vi "App - analyze RUS V6.vi"() -> ()   [LabVIEW 2021] (continued)
"z (pi/2)"=0.0+0.0i, "z center"=0.0+0.0i, "z(0)"=0.0+0.0i, "radius"=0.0}}, "timestamp(min)"=2847.0166666656733, "timestamp"=timestamp(3493898642 s since 1904-01-01), "Magn Field(T)"=0.0}, {"temperature"=14.778, "lorentzian"={"A (VHz)"=0.0, "ω (Hz)"=0.0, "Γ (Hz)"=0.0, "φ (rad)"=0.0, "Q"=0.0, "Norm  Ampl"=0.0, "z∞ (V)"=0.0+0.0i, "4corners"={"z (-pi/2)"=0.0+0.0i, "z(inf)"=0.0+0.0i, "z (pi/2)"=0.0+0.0i, "z center"=0.0+0.0i, "z(0)"=0.0+0.0i, "radius"=0.0}}, "timestamp(min)"=2848.333333335817, "timestamp"=timestamp(3493898721 s since 1904-01-01), "Magn Field(T)"=0.0}, {"temperature"=14.778, "lorentzian"={"A (VHz)"=0.0, "ω (Hz)"=0.0, "Γ (Hz)"=0.0, "φ (rad)"=0.0, "Q"=0.0, "Norm  Ampl"=0.0, "z∞ (V)"=0.0+0.0i, "4corners"={"z (-pi/2)"=0.0+0.0i, "z(inf)"=0.0+0.0i, "z (pi/2)"=0.0+0.0i, "z center"=0.0+0.0i, "z(0)"=0.0+0.0i, "radius"=0.0}}, "timestamp(min)"=2849.666666664183, "timestamp"=timestamp(3493898801 s since 1904-01-01), "Magn Field(T)"=0.0}, {"temperature"=14.784, "lorentzian"={"A (VHz)"=0.0, "ω (Hz)"=0.0, "Γ (Hz)"=0.0, "φ (rad)"=0.0, "Q"=0.0, "Norm  Ampl"=0.0, "z∞ (V)"=0.0+0.0i, "4corners"={"z (-pi/2)"=0.0+0.0i, "z(inf)"=0.0+0.0i, "z (pi/2)"=0.0+0.0i, "z center"=0.0+0.0i, "z(0)"=0.0+0.0i, "radius"=0.0}}, "timestamp(min)"=2850.9833333343267, "timestamp"=timestamp(3493898880 s since 1904-01-01), "Magn Field(T)"=0.0}, {"temperature"=14.784, "lorentzian"={"A (VHz)"=0.0, "ω (Hz)"=0.0, "Γ (Hz)"=0.0, "φ (rad)"=0.0, "Q"=0.0, "Norm  Ampl"=0.0, "z∞ (V)"=0.0+0.0i, "4corners"={"z (-pi/2)"=0.0+0.0i, "z(inf)"=0.0+0.0i, "z (pi/2)"=0.0+0.0i, "z center"=0.0+0.0i, "z(0)"=0.0+0.0i, "radius"=0.0}}, "timestamp(min)"=2852.3000000044703, "timestamp"=timestamp(3493898959 s since 1904-01-01), "Magn Field(T)"=0.0}, {"temperature"=14.784, "lorentzian"={"A (VHz)"=0.0, "ω (Hz)"=0.0, "Γ (Hz)"=0.0, "φ (rad)"=0.0, "Q"=0.0, "Norm  Ampl"=0.0, "z∞ (V)"=0.0+0.0i, "4corners"={"z (-pi/2)"=0.0+0.0i, "z(inf)"=0.0+0.0i, "z (pi/2)"=0.0+0.0i, "z center"=0.0+0.0i, "z(0)"=0.0+0.0i, "radius"=0.0}}, "timestamp(min)"=2853.6333333328366, "timestamp"=timestamp(3493899039 s since 1904-01-01), "Magn Field(T)"=0.0}, {"temperature"=14.789, "lorentzian"={"A (VHz)"=0.0, "ω (Hz)"=0.0, "Γ (Hz)"=0.0, "φ (rad)"=0.0, "Q"=0.0, "Norm  Ampl"=0.0, "z∞ (V)"=0.0+0.0i, "4corners"={"z (-pi/2)"=0.0+0.0i, "z(inf)"=0.0+0.0i, "z (pi/2)"=0.0+0.0i, "z center"=0.0+0.0i, "z(0)"=0.0+0.0i, "radius"=0.0}}, "timestamp(min)"=2854.9500000029802, "timestamp"=timestamp(3493899118 s since 1904-01-01), "Magn Field(T)"=0.0}, {"temperature"=14.788, "lorentzian"={"A (VHz)"=0.0, "ω (Hz)"=0.0, "Γ (Hz)"=0.0, "φ (rad)"=0.0, "Q"=0.0, "Norm  Ampl"=0.0, "z∞ (V)"=0.0+0.0i, "4corners"={"z (-pi/2)"=0.0+0.0i, "z(inf)"=0.0+0.0i, "z (pi/2)"=0.0+0.0i, "z center"=0.0+0.0i, "z(0)"=0.0+0.0i, "radius"=0.0}}, "timestamp(min)"=2856.2833333313465, "timestamp"=timestamp(3493899198 s since 1904-01-01), "Magn Field(T)"=0.0}, {"temperature"=14.791, "lorentzian"={"A (VHz)"=0.0, "ω (Hz)"=0.0, "Γ (Hz)"=0.0, "φ (rad)"=0.0, "Q"=0.0, "Norm  Ampl"=0.0, "z∞ (V)"=0.0+0.0i, "4corners"={"z (-pi/2)"=0.0+0.0i, "z(inf)"=0.0+0.0i, "z (pi/2)"=0.0+0.0i, "z center"=0.0+0.0i, "z(0)"=0.0+0.0i, "radius"=0.0}}, "timestamp(min)"=2857.60000000149, "timestamp"=timestamp(3493899277 s since 1904-01-01), "Magn Field(T)"=0.0}, {"temperature"=14.793, "lorentzian"={"A (VHz)"=0.0, "ω (Hz)"=0.0, "Γ (Hz)"=0.0, "φ (rad)"=0.0, "Q"=0.0, "Norm  Ampl"=0.0, "z∞ (V)"=0.0+0.0i, "4corners"={"z (-pi/2)"=0.0+0.0i, "z(inf)"=0.0+0.0i, "z (pi/2)"=0.0+0.0i, "z center"=0.0+0.0i, "z(0)"=0.0+0.0i, "radius"=0.0}}, "timestamp(min)"=2858.916666664183, "timestamp"=timestamp(3493899356 s since 1904-01-01), "Magn Field(T)"=0.0}, {"temperature"=14.796, "lorentzian"={"A (VHz)"=0.0, "ω (Hz)"=0.0, "Γ (Hz)"=0.0, "φ (rad)"=0.0, "Q"=0.0, "Norm  Ampl"=0.0, "z∞ (V)"=0.0+0.0i, "4corners"={"z (-pi/2)"=0.0+0.0i, "z(inf)"=0.0+0.0i, "z (pi/2)"=0.0+0.0i, "z center"=0.0+0.0i, "z(0)"=0.0+0.0i, "radius"=0.0}}, "timestamp(min)"=2860.25, "timestamp"=timestamp(3493899436 s since 1904-01-01), "Magn Field(T)"=0.0}, {"temperature"=14.797, "lorentzian"={"A (VHz)"=0.0, "ω (Hz)"=0.0, "Γ (Hz)"=0.0, "φ (rad)"=0.0, "Q"=0.0, "Norm  Ampl"=0.0, "z∞ (V)"=0.0+0.0i, "4corners"={"z (-pi/2)"=0.0+0.0i, "z(inf)"=0.0+0.0i, "z (pi/2)"=0.0+0.0i, "z center"=0.0+0.0i, "z(0)"=0.0+0.0i, "radius"=0.0}}, "timestamp(min)"=2861.5666666701436, "timestamp"=timestamp(3493899515 s since 1904-01-01), "Magn Field(T)"=0.0}, {"temperature"=14.8, "lorentzian"={"A (VHz)"=0.0, "ω (Hz)"=0.0, "Γ (Hz)"=0.0, "φ (rad)"=0.0, "Q"=0.0, "Norm  Ampl"=0.0, "z∞ (V)"=0.0+0.0i, "4corners"={"z (-pi/2)"=0.0+0.0i, "z(inf)"=0.0+0.0i, "z (pi/2)"=0.0+0.0i, "z center"=0.0+0.0i, "z(0)"=0.0+0.0i, "radius"=0.0}}, "timestamp(min)"=2862.8833333328366, "timestamp"=timestamp(3493899594 s since 1904-01-01), "Magn Field(T)"=0.0}, {"temperature"=14.807, "lorentzian"={"A (VHz)"=0.0, "ω (Hz)"=0.0, "Γ (Hz)"=0.0, "φ (rad)"=0.0, "Q"=0.0, "Norm  Ampl"=0.0, "z∞ (V)"=0.0+0.0i, "4corners"={"z (-pi/2)"=0.0+0.0i, "z(inf)"=0.0+0.0i, "z (pi/2)"=0.0+0.0i, "z center"=0.0+0.0i, "z(0)"=0.0+0.0i, "radius"=0.0}}, "timestamp(min)"=2864.2166666686535, "timestamp"=timestamp(3493899674 s since 1904-01-01), "Magn Field(T)"=0.0}, {"temperature"=14.806, "lorentzian"={"A (VHz)"=0.0, "ω (Hz)"=0.0, "Γ (Hz)"=0.0, "φ (rad)"=0.0, "Q"=0.0, "Norm  Ampl"=0.0, "z∞ (V)"=0.0+0.0i, "4corners"={"z (-pi/2)"=0.0+0.0i, "z(inf)"=0.0+0.0i, "z (pi/2)"=0.0+0.0i, "z center"=0.0+0.0i, "z(0)"=0.0+0.0i, "radius"=0.0}}, "timestamp(min)"=2865.5333333313465, "timestamp"=timestamp(3493899753 s since 1904-01-01), "Magn Field(T)"=0.0}, {"temperature"=14.808, "lorentzian"={"A (VHz)"=0.0, "ω (Hz)"=0.0, "Γ (Hz)"=0.0, "φ (rad)"=0.0, "Q"=0.0, "Norm  Ampl"=0.0, "z∞ (V)"=0.0+0.0i, "4corners"={"z (-pi/2)"=0.0+0.0i, "z(inf)"=0.0+0.0i, "z (pi/2)"=0.0+0.0i, "z center"=0.0+0.0i, "z(0)"=0.0+0.0i, "radius"=0.0}}, "timestamp(min)"=2866.8666666671634, "timestamp"=timestamp(3493899833 s since 1904-01-01), "Magn Field(T)"=0.0}, {"temperature"=14.812, "lorentzian"={"A (VHz)"=0.0, "ω (Hz)"=0.0, "Γ (Hz)"=0.0, "φ (rad)"=0.0, "Q"=0.0, "Norm  Ampl"=0.0, "z∞ (V)"=0.0+0.0i, "4corners"={"z (-pi/2)"=0.0+0.0i, "z(inf)"=0.0+0.0i, "z (pi/2)"=0.0+0.0i, "z center"=0.0+0.0i, "z(0)"=0.0+0.0i, "radius"=0.0}}, "timestamp(min)"=2868.183333337307, "timestamp"=timestamp(3493899912 s since 1904-01-01), "Magn Field(T)"=0.0}, {"temperature"=14.814, "lorentzian"={"A (VHz)"=0.0, "ω (Hz)"=0.0, "Γ (Hz)"=0.0, "φ (rad)"=0.0, "Q"=0.0, "Norm  Ampl"=0.0, "z∞ (V)"=0.0+0.0i, "4corners"={"z (-pi/2)"=0.0+0.0i, "z(inf)"=0.0+0.0i, "z (pi/2)"=0.0+0.0i, "z center"=0.0+0.0i, "z(0)"=0.0+0.0i, "radius"=0.0}}, "timestamp(min)"=2869.5, "timestamp"=timestamp(3493899991 s since 1904-01-01), "Magn Field(T)"=0.0}, {"temperature"=14.82, "lorentzian"={"A (VHz)"=0.0, "ω (Hz)"=0.0, "Γ (Hz)"=0.0, "φ (rad)"=0.0, "Q"=0.0, "Norm  Ampl"=0.0, "z∞ (V)"=0.0+0.0i, "4corners"={"z (-pi/2)"=0.0+0.0i, "z(inf)"=0.0+0.0i, "z (pi/2)"=0.0+0.0i, "z center"=0.0+0.0i, "z(0)"=0.0+0.0i, "radius"=0.0}}, "timestamp(min)"=2870.833333335817, "timestamp"=timestamp(3493900071 s since 1904-01-01), "Magn Field(T)"=0.0}, {"temperature"=14.816, "lorentzian"={"A (VHz)"=0.0, "ω (Hz)"=0.0, "Γ (Hz)"=0.0, "φ (rad)"=0.0, "Q"=0.0, "Norm  Ampl"=0.0, "z∞ (V)"=0.0+0.0i, "4corners"={"z (-pi/2)"=0.0+0.0i, "z(inf)"=0.0+0.0i, "z (pi/2)"=0.0+0.0i, "z center"=0.0+0.0i, "z(0)"=0.0+0.0i, "radius"=0.0}}, "timestamp(min)"=2872.14999999851, "timestamp"=timestamp(3493900150 s since 1904-01-01), "Magn Field(T)"=0.0}] {"lorentzian"."z∞ (V)" format="%#_4p"; "lorentzian"."Q" format="%#_4p"; "lorentzian"."φ (rad)" format="%#_3p"; "lorentzian"."Γ (Hz)" format="%#_5p"; "lorentzian"."ω (Hz)" format="%#_9p"; "lorentzian"."A (VHz)" format="%#_3p"}
  in  "cursor bracket: fragment":T24={"left"=663.5468604577721, "right "=663.8468604577721, "center"=663.6968604577721, "window"=0.30000000000000004, "cursors"=[0, 1, 2], "relative"=0, "absolute"=0, "fixed vertical offset"=0.0, "vertical offset"=0.0, "skew"=0.0, "default window frac"=0.1, "kind"=enum."symmetric", "skew.left"=0.5, "skew.right"=0.5, "Plot ref"=refnum, "wing order"=enum."back"}
  in  "cursor bracket: All, data window":T24={"left"=655.6615812868605, "right "=667.1582032202367, "center"=663.6968604577721, "window"=11.496621933376199, "cursors"=[0, 1, 2], "relative"=0, "absolute"=0, "fixed vertical offset"=0.0, "vertical offset"=0.0, "skew"=-0.3978504672897196, "default window frac"=0.1, "kind"=enum."skewed", "skew.left"=0.6989252336448598, "skew.right"=0.3010747663551402, "Plot ref"=refnum, "wing order"=enum."back"}
  in  "cursor bracket: All,  zoom":T24={"left"=842.6955942299186, "right "=2207.477971149593, "center"=1525.0867826897559, "window"=1364.7823769196746, "cursors"=[3, 4, 5], "relative"=0, "absolute"=0, "fixed vertical offset"=0.0, "vertical offset"=0.0, "skew"=0.0, "default window frac"=0.1, "kind"=enum."symmetric", "skew.left"=0.5, "skew.right"=0.5, "Plot ref"=refnum, "wing order"=enum."back"}
  in  "plot scale: Geometry":T28={"Plot Ref"=refnum, "center"=0.0, "delta"=100.0, "mode"=enum."no filter", "scale cursor index"=10, "history"=100.0, "history array"=[0.5, 0.5, 0.5, 0.5, 0.5, 0.5, 0.5, 0.5, 0.5, 0.5, 0.5, 0.5, 0.5, 0.5, 0.5, 0.5, 0.5, 0.5, 0.5, 0.5, 0.5, 0.5, 0.5, 0.5, 0.5, 0.5, 0.5, 0.5, 0.5, 0.5, 0.5, 0.5, 0.5, 0.5, 0.5, 0.5, 0.5, 0.5, 0.5, 0.5, 0.5, 0.5, 0.5, 0.5, 0.5, 0.5, 0.5, 0.5, 0.5, 0.5, 0.5, 0.5, 0.5, 0.5, 0.5, 0.5, 0.5, 0.5, 0.5, 0.5, 0.5, 0.5, 0.5, 0.5, 0.5, 0.5, 0.5, 0.5, 0.5, 0.5, 0.5, 0.5, 0.5, 0.5, 0.5, 0.5, 0.5, 0.5, 0.5, 0.5, 0.5, 0.5, 0.5, 0.5, 0.5, 0.5, 0.5, 0.5, 0.5, 0.5, 0.5, 0.5, 0.5, 0.5, 0.5, 0.5, 0.5, 0.5, 0.5, 0.5]}
  in  "plot scale: delta f":T28={"Plot Ref"=refnum, "center"=0.0, "delta"=60.0, "mode"=enum."no filter", "scale cursor index"=10, "history"=100.0, "history array"=[0.5, 0.5, 0.5, 0.5, 0.5, 0.5, 0.5, 0.5, 0.5, 0.5, 0.5, 0.5, 0.5, 0.5, 0.5, 0.5, 0.5, 0.5, 0.5, 0.5, 0.5, 0.5, 0.5, 0.5, 0.5, 0.5, 0.5, 0.5, 0.5, 0.5, 0.5, 0.5, 0.5, 0.5, 0.5, 0.5, 0.5, 0.5, 0.5, 0.5, 0.5, 0.5, 0.5, 0.5, 0.5, 0.5, 0.5, 0.5, 0.5, 0.5, 0.5, 0.5, 0.5, 0.5, 0.5, 0.5, 0.5, 0.5, 0.5, 0.5, 0.5, 0.5, 0.5, 0.5, 0.5, 0.5, 0.5, 0.5, 0.5, 0.5, 0.5, 0.5, 0.5, 0.5, 0.5, 0.5, 0.5, 0.5, 0.5, 0.5, 0.5, 0.5, 0.5, 0.5, 0.5, 0.5, 0.5, 0.5, 0.5, 0.5, 0.5, 0.5, 0.5, 0.5, 0.5, 0.5, 0.5, 0.5, 0.5, 0.5]}
  in  "plot scale: frequency vs T":T28={"Plot Ref"=refnum, "center"=0.0, "delta"=100.0, "mode"=enum."no filter", "scale cursor index"=10, "history"=100.0, "history array"=[0.5, 0.5, 0.5, 0.5, 0.5, 0.5, 0.5, 0.5, 0.5, 0.5, 0.5, 0.5, 0.5, 0.5, 0.5, 0.5, 0.5, 0.5, 0.5, 0.5, 0.5, 0.5, 0.5, 0.5, 0.5, 0.5, 0.5, 0.5, 0.5, 0.5, 0.5, 0.5, 0.5, 0.5, 0.5, 0.5, 0.5, 0.5, 0.5, 0.5, 0.5, 0.5, 0.5, 0.5, 0.5, 0.5, 0.5, 0.5, 0.5, 0.5, 0.5, 0.5, 0.5, 0.5, 0.5, 0.5, 0.5, 0.5, 0.5, 0.5, 0.5, 0.5, 0.5, 0.5, 0.5, 0.5, 0.5, 0.5, 0.5, 0.5, 0.5, 0.5, 0.5, 0.5, 0.5, 0.5, 0.5, 0.5, 0.5, 0.5, 0.5, 0.5, 0.5, 0.5, 0.5, 0.5, 0.5, 0.5, 0.5, 0.5, 0.5, 0.5, 0.5, 0.5, 0.5, 0.5, 0.5, 0.5, 0.5, 0.5]}
  in  "plot scale: All":T28={"Plot Ref"=refnum, "center"=0.0, "delta"=0.1, "mode"=enum."no filter", "scale cursor index"=10, "history"=100.0, "history array"=[0.5, 0.5, 0.5, 0.5, 0.5, 0.5, 0.5, 0.5, 0.5, 0.5, 0.5, 0.5, 0.5, 0.5, 0.5, 0.5, 0.5, 0.5, 0.5, 0.5, 0.5, 0.5, 0.5, 0.5, 0.5, 0.5, 0.5, 0.5, 0.5, 0.5, 0.5, 0.5, 0.5, 0.5, 0.5, 0.5, 0.5, 0.5, 0.5, 0.5, 0.5, 0.5, 0.5, 0.5, 0.5, 0.5, 0.5, 0.5, 0.5, 0.5, 0.5, 0.5, 0.5, 0.5, 0.5, 0.5, 0.5, 0.5, 0.5, 0.5, 0.5, 0.5, 0.5, 0.5, 0.5, 0.5, 0.5, 0.5, 0.5, 0.5, 0.5, 0.5, 0.5, 0.5, 0.5, 0.5, 0.5, 0.5, 0.5, 0.5, 0.5, 0.5, 0.5, 0.5, 0.5, 0.5, 0.5, 0.5, 0.5, 0.5, 0.5, 0.5, 0.5, 0.5, 0.5, 0.5, 0.5, 0.5, 0.5, 0.5]}
  in  "plot scale: Attenuation vs T":T28={"Plot Ref"=refnum, "center"=0.0, "delta"=50.0, "mode"=enum."no filter", "scale cursor index"=10, "history"=100.0, "history array"=[0.5, 0.5, 0.5, 0.5, 0.5, 0.5, 0.5, 0.5, 0.5, 0.5, 0.5, 0.5, 0.5, 0.5, 0.5, 0.5, 0.5, 0.5, 0.5, 0.5, 0.5, 0.5, 0.5, 0.5, 0.5, 0.5, 0.5, 0.5, 0.5, 0.5, 0.5, 0.5, 0.5, 0.5, 0.5, 0.5, 0.5, 0.5, 0.5, 0.5, 0.5, 0.5, 0.5, 0.5, 0.5, 0.5, 0.5, 0.5, 0.5, 0.5, 0.5, 0.5, 0.5, 0.5, 0.5, 0.5, 0.5, 0.5, 0.5, 0.5, 0.5, 0.5, 0.5, 0.5, 0.5, 0.5, 0.5, 0.5, 0.5, 0.5, 0.5, 0.5, 0.5, 0.5, 0.5, 0.5, 0.5, 0.5, 0.5, 0.5, 0.5, 0.5, 0.5, 0.5, 0.5, 0.5, 0.5, 0.5, 0.5, 0.5, 0.5, 0.5, 0.5, 0.5, 0.5, 0.5, 0.5, 0.5, 0.5, 0.5]}
  in  "9w folder path":path=path "D:/Data/Ultrasound/LSCO/LSCO22__130814c/5_Cooling_2nd_try/9w"
  in  "help toggle":bool=TRUE
  in  "cursor bracket: All,  show":T24={"left"=1443.1667294308304, "right "=1448.993434554408, "center"=1446.0800819926192, "window"=5.826705123577359, "cursors"=[6, 7, 8], "relative"=0, "absolute"=0, "fixed vertical offset"=0.0, "vertical offset"=0.0, "skew"=0.0, "default window frac"=0.1, "kind"=enum."symmetric", "skew.left"=0.5, "skew.right"=0.5, "Plot ref"=refnum, "wing order"=enum."back"}
  in  "plot scale: df/dT":T28={"Plot Ref"=refnum, "center"=0.0, "delta"=60.0, "mode"=enum."no filter", "scale cursor index"=10, "history"=100.0, "history array"=[0.5, 0.5, 0.5, 0.5, 0.5, 0.5, 0.5, 0.5, 0.5, 0.5, 0.5, 0.5, 0.5, 0.5, 0.5, 0.5, 0.5, 0.5, 0.5, 0.5, 0.5, 0.5, 0.5, 0.5, 0.5, 0.5, 0.5, 0.5, 0.5, 0.5, 0.5, 0.5, 0.5, 0.5, 0.5, 0.5, 0.5, 0.5, 0.5, 0.5, 0.5, 0.5, 0.5, 0.5, 0.5, 0.5, 0.5, 0.5, 0.5, 0.5, 0.5, 0.5, 0.5, 0.5, 0.5, 0.5, 0.5, 0.5, 0.5, 0.5, 0.5, 0.5, 0.5, 0.5, 0.5, 0.5, 0.5, 0.5, 0.5, 0.5, 0.5, 0.5, 0.5, 0.5, 0.5, 0.5, 0.5, 0.5, 0.5, 0.5, 0.5, 0.5, 0.5, 0.5, 0.5, 0.5, 0.5, 0.5, 0.5, 0.5, 0.5, 0.5, 0.5, 0.5, 0.5, 0.5, 0.5, 0.5, 0.5, 0.5]}
  in  "plots: filter related":T29
  in  "plot scale: Attenuation vs H":T28={"Plot Ref"=refnum, "center"=0.0, "delta"=50.0, "mode"=enum."no filter", "scale cursor index"=10, "history"=100.0, "history array"=[0.5, 0.5, 0.5, 0.5, 0.5, 0.5, 0.5, 0.5, 0.5, 0.5, 0.5, 0.5, 0.5, 0.5, 0.5, 0.5, 0.5, 0.5, 0.5, 0.5, 0.5, 0.5, 0.5, 0.5, 0.5, 0.5, 0.5, 0.5, 0.5, 0.5, 0.5, 0.5, 0.5, 0.5, 0.5, 0.5, 0.5, 0.5, 0.5, 0.5, 0.5, 0.5, 0.5, 0.5, 0.5, 0.5, 0.5, 0.5, 0.5, 0.5, 0.5, 0.5, 0.5, 0.5, 0.5, 0.5, 0.5, 0.5, 0.5, 0.5, 0.5, 0.5, 0.5, 0.5, 0.5, 0.5, 0.5, 0.5, 0.5, 0.5, 0.5, 0.5, 0.5, 0.5, 0.5, 0.5, 0.5, 0.5, 0.5, 0.5, 0.5, 0.5, 0.5, 0.5, 0.5, 0.5, 0.5, 0.5, 0.5, 0.5, 0.5, 0.5, 0.5, 0.5, 0.5, 0.5, 0.5, 0.5, 0.5, 0.5]}
  in  "plot scale: frequency vs H":T28={"Plot Ref"=refnum, "center"=0.0, "delta"=50.0, "mode"=enum."no filter", "scale cursor index"=10, "history"=100.0, "history array"=[0.5, 0.5, 0.5, 0.5, 0.5, 0.5, 0.5, 0.5, 0.5, 0.5, 0.5, 0.5, 0.5, 0.5, 0.5, 0.5, 0.5, 0.5, 0.5, 0.5, 0.5, 0.5, 0.5, 0.5, 0.5, 0.5, 0.5, 0.5, 0.5, 0.5, 0.5, 0.5, 0.5, 0.5, 0.5, 0.5, 0.5, 0.5, 0.5, 0.5, 0.5, 0.5, 0.5, 0.5, 0.5, 0.5, 0.5, 0.5, 0.5, 0.5, 0.5, 0.5, 0.5, 0.5, 0.5, 0.5, 0.5, 0.5, 0.5, 0.5, 0.5, 0.5, 0.5, 0.5, 0.5, 0.5, 0.5, 0.5, 0.5, 0.5, 0.5, 0.5, 0.5, 0.5, 0.5, 0.5, 0.5, 0.5, 0.5, 0.5, 0.5, 0.5, 0.5, 0.5, 0.5, 0.5, 0.5, 0.5, 0.5, 0.5, 0.5, 0.5, 0.5, 0.5, 0.5, 0.5, 0.5, 0.5, 0.5, 0.5]}
  out "script event":string
  in  "tfolder":T30={"tfolder path"=path "D:/Data/Ultrasound/LSCO/LSCO22__130814c/5_Cooling_2nd_try", "9folder path"=path "D:/Data/Ultrasound/LSCO/LSCO22__130814c/5_Cooling_2nd_try/9w", "tfolder  -  file array"=[{"timestamp from"=43.433333337306976, "timestamp to"=2233.166666664183, " index  from"=17, "index to"=1672, "active"=TRUE}, {"timestamp from"=2241.10000000149, "timestamp to"=2399.8666666671634, " index  from"=1678, "index to"=1798, "active"=TRUE}, {"timestamp from"=2423.683333337307, "timestamp to"=2870.833333335817, " index  from"=1816, "index to"=2154, "active"=TRUE}], "from index array"=[17, 1678, 1816], "timestamp array"=[43.433333337306976, 2241.10000000149, 2423.683333337307]}
  in  "Tab : dummy":enum32{"Page 1", "Page 2"}(tab)
  out "Plot: dTemp/dTime":cluster{dbl[], dbl[]}[](graph)
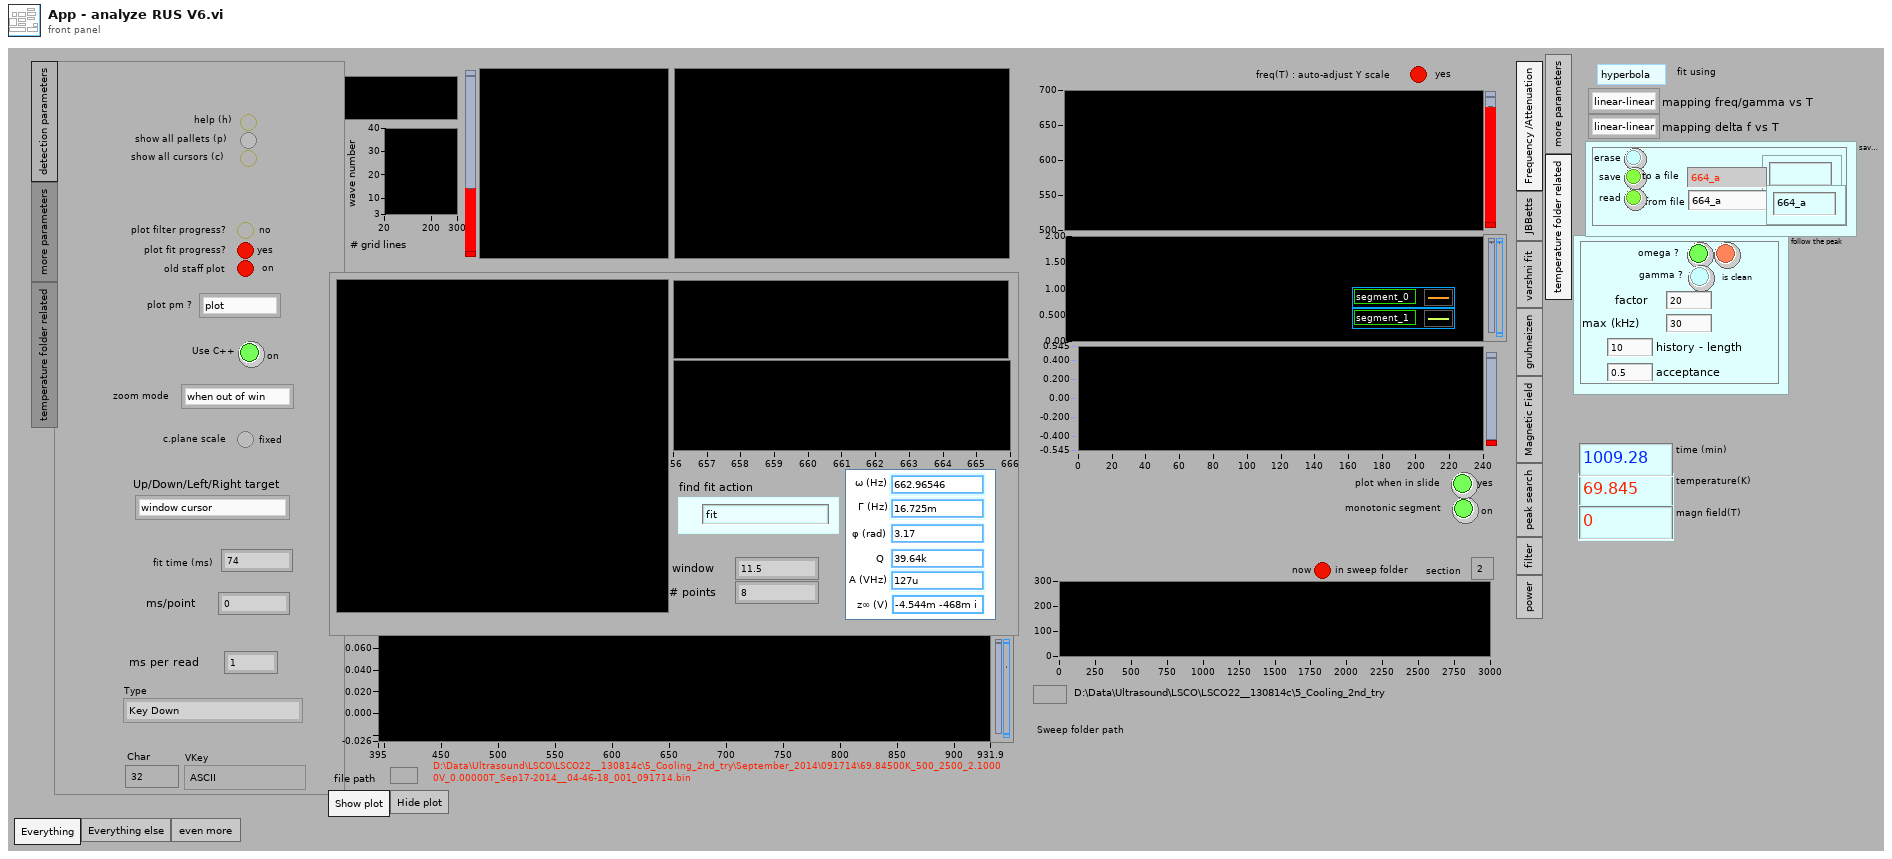
[diagram p1: front panel]
types:
  T1 = enum32{"more parameters", "temperature folder related"}
  T2 = typedef "read scan file control.ctl" = cluster{"# columns":i32, "create bin file":bool, "do not filter":bool, "normalize phase":bool, "read freq units":enum16{"kHz", "Hz"}}
  T3 = enum16{"linear-linear", "log-linear", "linear-log", "log-log"}
  T4 = typedef "old slider control.ctl" = cluster{"in slide":bool, "direction":bool, "start ":bool, "stop":bool, "next":bool}
  T5 = typedef "fit function selector control.ctl" = enum16{"linear", "varshni", "varshni5", "LogMinusT", "hyperbola", "einstein", "sine", "sine2theta", "cos2theta"}
  T6 = typedef "freq file read-write control.ctl" = cluster{"write to a file list":u16, "from file ":string, "erase":bool, "load":bool, "save":bool, "to a file ":string, "read from file list":u16}
  T7 = typedef "follow the peak control.ctl" = cluster{"factor":dbl, "omega ?":bool, "gamma ?":bool, "max (kHz)":dbl, "is clean":bool, "acceptance":dbl, "history - length":i32}
  T8 = enum32{"Everything", "Everything else", "even more "}
  T9 = enum32{"Frequency /Attenuation", "JBBetts", "varshni fit ", "gruhneizen", "Magnetic Field", "peak search", "filter", "power"}
  T10 = typedef "scale - offset gauge.ctl" = cluster{"scale offset":dbl, "scale range":dbl}
  T11 = typedef "lorentzian.ctl" = cluster{"A (VHz)":dbl, "ω (Hz)":dbl, "Γ (Hz)":dbl, "φ (rad)":dbl, "Q":dbl, "Norm  Ampl":dbl, "z∞ (V)":cdb, "4corners":T12}
  T12 = typedef "circle corners.ctl" = cluster{"z (-pi/2)":cdb, "z(inf)":cdb, "z (pi/2)":cdb, "z center":cdb, "z(0)":cdb, "radius":dbl}
  T13 = typedef "find peak action.ctl" = enum16{"empty", "-find center", "-mapping", "fit", "-shake it one", "bbb", "-update pond", "move z(center)", "move z(inf)", "update pond", "fancy fit one", "fragment window moves", "-shake it two", "fancy fit two", "pm fit"}
  T14 = cluster{"omega out":dbl[], "win omega out":dbl[]}
  T15 = typedef "peak -- parameters -- complex fit.ctl" = cluster{"main VI path":path, "scale factor":dbl, "# of grid points":i32, "parameters: wavepacket":T16, "span":dbl, "interference ?":enum16{"cp z center", "pm zcenter", "fancy"}, "filter method":T17}
  T16 = typedef "wavepacket.ctl" = cluster{"R":dbl, "wave number":dbl, "delta k":dbl, "radii vector":dbl[], "radial section":cdb[], "wave vector":dbl, "wavepacket is":bool}
  T17 = typedef "filter method control.ctl" = enum16{"four", "five", "one", "two", "three", "zero", "minus one", "minus two"}
  T18 = enum32{"detection parameters", "more parameters", "temperature folder related"}
  T19 = typedef "eventvkey.ctl" = enum16{"ASCII", "Enter", "Return", "Shift", "Ctrl", "Alt", "Cmd", "Opt", "Caps", "NumLock", "Clear", "Break", "Up", "Down", "Left", "Right", "Insert", "Delete", "Home", "End", "PageUp", "PageDown", "Escape", "Help", "Pause", "ScrollLock", "F1", "F2", "F3", "F4", "F5", "F6", "F7", "F8", "F9", "F10", "F11", "F12", "F13", "F14", "F15", "F16", "F17", "F18", "F19", "F20", "F21", "F22", "F23", "F24", "Play", "VolumeUp", "VolumeDown", "Mute", "Two Byte Char"}
  T20 = typedef "lveventtype.ctl" = enum32{"Null", "Timeout", "Annotation Menu Selection", "Annotation Menu Selection?", "App Instance Close", "App Instance Close?", "Autoscale Range Change", "Bookmark Info Change", "Cell Edit", "Cell Edit?", "Cursor Grab", "Cursor Grab?", "Cursor Menu Selection", "Cursor Menu Selection?", "Cursor Move", "Cursor Release", "Data Change", "Direction Change", "Display State Change", "Drag Ended", "Drag Enter", "Drag Leave", "Drag Over", "Drag Source Update", "Drag Starting", "Drag Starting?", "Drop", "Exec State Change", "Key Down", "Key Down?", "Key Repeat", "Key Repeat?", "Key Up", "Listbox Double Click", "Menu Activation?", "Menu Selection (App)", "Menu Selection? (App)", "Menu Selection (User)", "Mouse Down", "Mouse Down?", "Mouse Enter", "Mouse Leave", "Mouse Move", "Mouse Up", "Mouse Wheel", "NI Security User Change (App)", "Pane Size", "Panel Close", "Panel Close?", "Panel Resize", "Plot Attribute Change", "Scale Range Change", "Shortcut Menu Activation?", "Shortcut Menu Selection (App)", "Shortcut Menu Selection? (App)", "Shortcut Menu Selection (User)", "Tree Double Click", "Tree Drag", "Tree Drag?", "Tree Drop", "Tree Drop?", "Tree Item Close", "Tree Item Close?", "Tree Item Open", "Tree Item Open?", "User Event", "Value Change"}
  T21 = typedef "single fit parameters.ctl" = cluster{"number of 2D grid points":i32, "# of points in pond":i32, "# of points in window":i32, "decimation threshold":i32, "normalization factor":dbl, "pond scale factor ":dbl, "normalized z":cdb[], "decimated z":cdb[], "decimated omega":dbl[], "omega in window":dbl[], "z in window":cdb[], "data center":cdb, "inverse":cdb[], "linear ":cdb[], "omega around":dbl[], "phase around center":dbl[], "fit for phase around senter ":dbl[], "three points":cluster{dbl[], dbl[]}, "max omega":dbl, "min omega":dbl, "dz/domega":cdb[]}
  T22 = typedef "omega map parameters.ctl" = cluster{"map method":enum16{"simple", "less trivial", "around center", "geometry"}, "2:window factor":i32, "left":dbl, "right":dbl, "omega":dbl, "gamma":dbl, "theta0":dbl, "use points":enum16{"all in window", "decimated"}, "z(inf) method":enum16{"median", "method 2", "histogram"}}
  T23 = cluster{"waveform  radial -  radii vector":dbl[], dbl[]}[]
  T24 = typedef "cursor winow.ctl" = cluster{"left":dbl, "right ":dbl, "center":dbl, "window":dbl, "cursors":i32[], "relative":i32, "absolute":i32, "fixed vertical offset":dbl, "vertical offset":dbl, "skew":dbl, "default window frac":dbl, "kind":enum16{"symmetric", "skewed", "fancy"}, "skew.left":dbl, "skew.right":dbl, "Plot ref":refnum<vi>, "wing order":enum16{"forw", "back"}}
  T25 = typedef "complex region.ctl" = cluster{"max re":dbl, "min re":dbl, "max im":dbl, "min im":dbl, "delta re":dbl, "delta im":dbl, "center re":dbl, "delta  z":cdb, "center im":dbl, "center z":cdb, "d im":dbl, "d re":dbl, "d z":cdb}
  T26 = typedef "sweep file name.ctl" = cluster{"temperature":dbl, "temperature str":string, "file path":path, "last mod":timestamp, "file name str":string, "mod time(min)":dbl, "file format":enum16{"", "ascii", "binary"}, "power(V)":dbl, "Magn Field(T) ":dbl}
  T27 = typedef "temperature sweep point.ctl" = cluster{"temperature":dbl, "lorentzian":T11, "timestamp(min)":dbl, "timestamp":timestamp, "Magn Field(T)":dbl}
  T28 = typedef "plot scale state.ctl" = cluster{"Plot Ref":refnum<vi>, "center":dbl, "delta":dbl, "mode":enum16{"no filter", "median", "liner fit on median"}, "scale cursor index":i32, "history":dbl, "history array":dbl[]}
  T29 = typedef "plot refs -- filter related.ctl" = cluster{"Plot: complex plane - filter":refnum<vi>, "Plot: dz/domega":refnum<vi>, "Plot: fragment filter":refnum<vi>, "Plot: win omega":refnum<vi>, "Plot: phase":refnum<vi>, "Plot: phase around center":refnum<vi>, "Plot: complex plane":refnum<vi>, "Plot: fragment":refnum<vi>}
  T30 = typedef "tfolder.ctl" = cluster{"tfolder path":path, "9folder path":path, "tfolder  -  file array":T31[], "from index array":i32[], "timestamp array":dbl[]}
  T31 = typedef "tfolder -- monotonic segment.ctl" = cluster{"timestamp from":dbl, "timestamp to":dbl, " index  from":i32, "index to":i32, "active":bool}
  T32 = typedef "slide action.ctl" = enum16{"start slide", "stop slide", "init", "check", "halt", "un-next", "next", "run", "slide UP", "slide DOWN"}
  T33 = typedef "follow the peak action.ctl" = enum16{"make clean", "make dirty", "follow the peak", "unfollow the peak", "follow gamma", "unfollow gamma", "check", "toggle omega", "toggle gamma"}
  T34 = typedef "cursor window action.ctl" = enum16{"balance", "h. offset change", "cursor moves", "change center", "change window", "init", "check", "reset", "set y to middle", "idle", "-write all Y", "-write left.X", "-write center.X", "-write right.X", "-write all X", "-change center", "-change window", "-change skew", "-read cursor 2", "-read cursor 1", "-read cursor 0", "-read all cursors", "-reset", "-read plot scale", "-set y to middle", "-Q: center.Y is visible", "-Q: window is visible", "-parse center.Y", "-right left from center", "-left move", "-right move", "-set center.Y", "-empty", "-set cursors to default", "-check", "-write center.Y", "-copy cursor 1", "-copy cursor 0", "-copy cursor 2", "move right", "move left", "shrink", "broaden", "skew up", "skew down", "-write plot scale", "zoom X", "change cen&win", "zoom to all data", "color--red", "color--green", "color--yellow", "read", "zoom out", "zoom in", "slide right", "slide left", "set range aspect ratio to 1", "move to window range", "--move to window range"}
  T35 = enum16{"normal", "alert", "fuzzy", "interesting", "boring", "colored"}
  T36 = typedef "save-read action.ctl" = enum16{"update save list", "update read list", "init", "check", "lookup read number", "lookup write number", "copy read from read ring", "saved file dirty", "saved file clean", "read file OK", "read file not OK", "nearest right", "nearest left", "increment read from", "copy read to save", "init save file", "erase event", "save event", "read event", "set save file", "decrement read from"}
  T37 = enum8{"Enabled", "Disabled", "Disabled and Grayed Out"}
  T38 = typedef "tale of three indices -- int -- control.ctl" = cluster{"left":i32, "center":i32, "right":i32, "right most":i32, "left most":i32, "window":i32, "max win factor":i32, "max win":i32, "min win":i32}
  T39 = cluster{"left":dbl, "right ":dbl, "center":dbl, "window":dbl, "cursors":i32[], "relative":i32, "absolute":i32, "fixed vertical offset":dbl, "vertical offset":dbl, "skew":dbl, "default window frac":dbl, "kind":enum16{"symmetric", "skewed", "fancy"}, "skew.left":dbl, "skew.right":dbl, "Plot ref":refnum<vi>, "wing order":enum16{"forw", "back"}}
  T40 = enum16{"new", "update range", "update monotonic pieces", "init", "check", "reset", ""}
  T41 = enum16{"mouse leave", "mouse enter", "mouse move", "manual zoom both", "manual zoom x", "manual zoom y"}
  T42 = typedef "LVRangeTypeDef.ctl" = cluster{"Minimum":dbl, "Maximum":dbl, "Increment":dbl, "Minor Increment":dbl, "Start":dbl}
  T43 = typedef "LVForegroundBackgroundColorsTypeDef.ctl" = cluster{"FG Color":u32, "BG Color":u32}
  T44 = typedef "LVCursorListTypeDef.ctl" = cluster{"Name":string, "Color":u32, "Style":u8, "Point Style":u8, "Name Visible":bool, "Allow Drag":bool, "Cursor Mode":u32, "Plot":i32, "Index":i32, "Position":cluster{"X":dbl, "Y":dbl}, "X Scale":u32, "Y Scale":u32, "Watch Plots":i32[], "Watch All Plots":bool, "Plot Area":i32, "Label Offset":cluster{"X":dbl, "Y":dbl}}[]
  T45 = cluster{"omega in window":dbl[], "phase around center":dbl[]}
  T46 = cluster{"omega in window":dbl[], "f(X,a)":dbl[]}[]
  T47 = cluster{"time points":dbl[], "temperature points":dbl[]}
  T48 = cluster{"time points":dbl[], "temperature points":dbl[]}[]
  T49 = cluster{"temperature points":dbl[], "derivative (kHz/min)":dbl[]}
  T50 = cluster{"time points":dbl[], "Magn Field points":dbl[]}
  T51 = cluster{"time points":dbl[], "frequency points":dbl[]}[]
  T52 = cluster{"temperature points":dbl[], "derivative (kHz/min)":dbl[]}[]
  T53 = cluster{"time points":dbl[], "Magn Field points":dbl[]}[]
  T54 = cluster{"Name":string, "Color":u32, "Style":u8, "Point Style":u8, "Name Visible":bool, "Allow Drag":bool, "Cursor Mode":u32, "Plot":i32, "Index":i32, "Position":cluster{"X":dbl, "Y":dbl}, "X Scale":u32, "Y Scale":u32, "Watch Plots":i32[], "Watch All Plots":bool, "Plot Area":i32, "Label Offset":cluster{"X":dbl, "Y":dbl}}
  T55 = typedef "LVPoint32TypeDef.ctl" = cluster{"Horizontal":i32, "Vertical":i32}
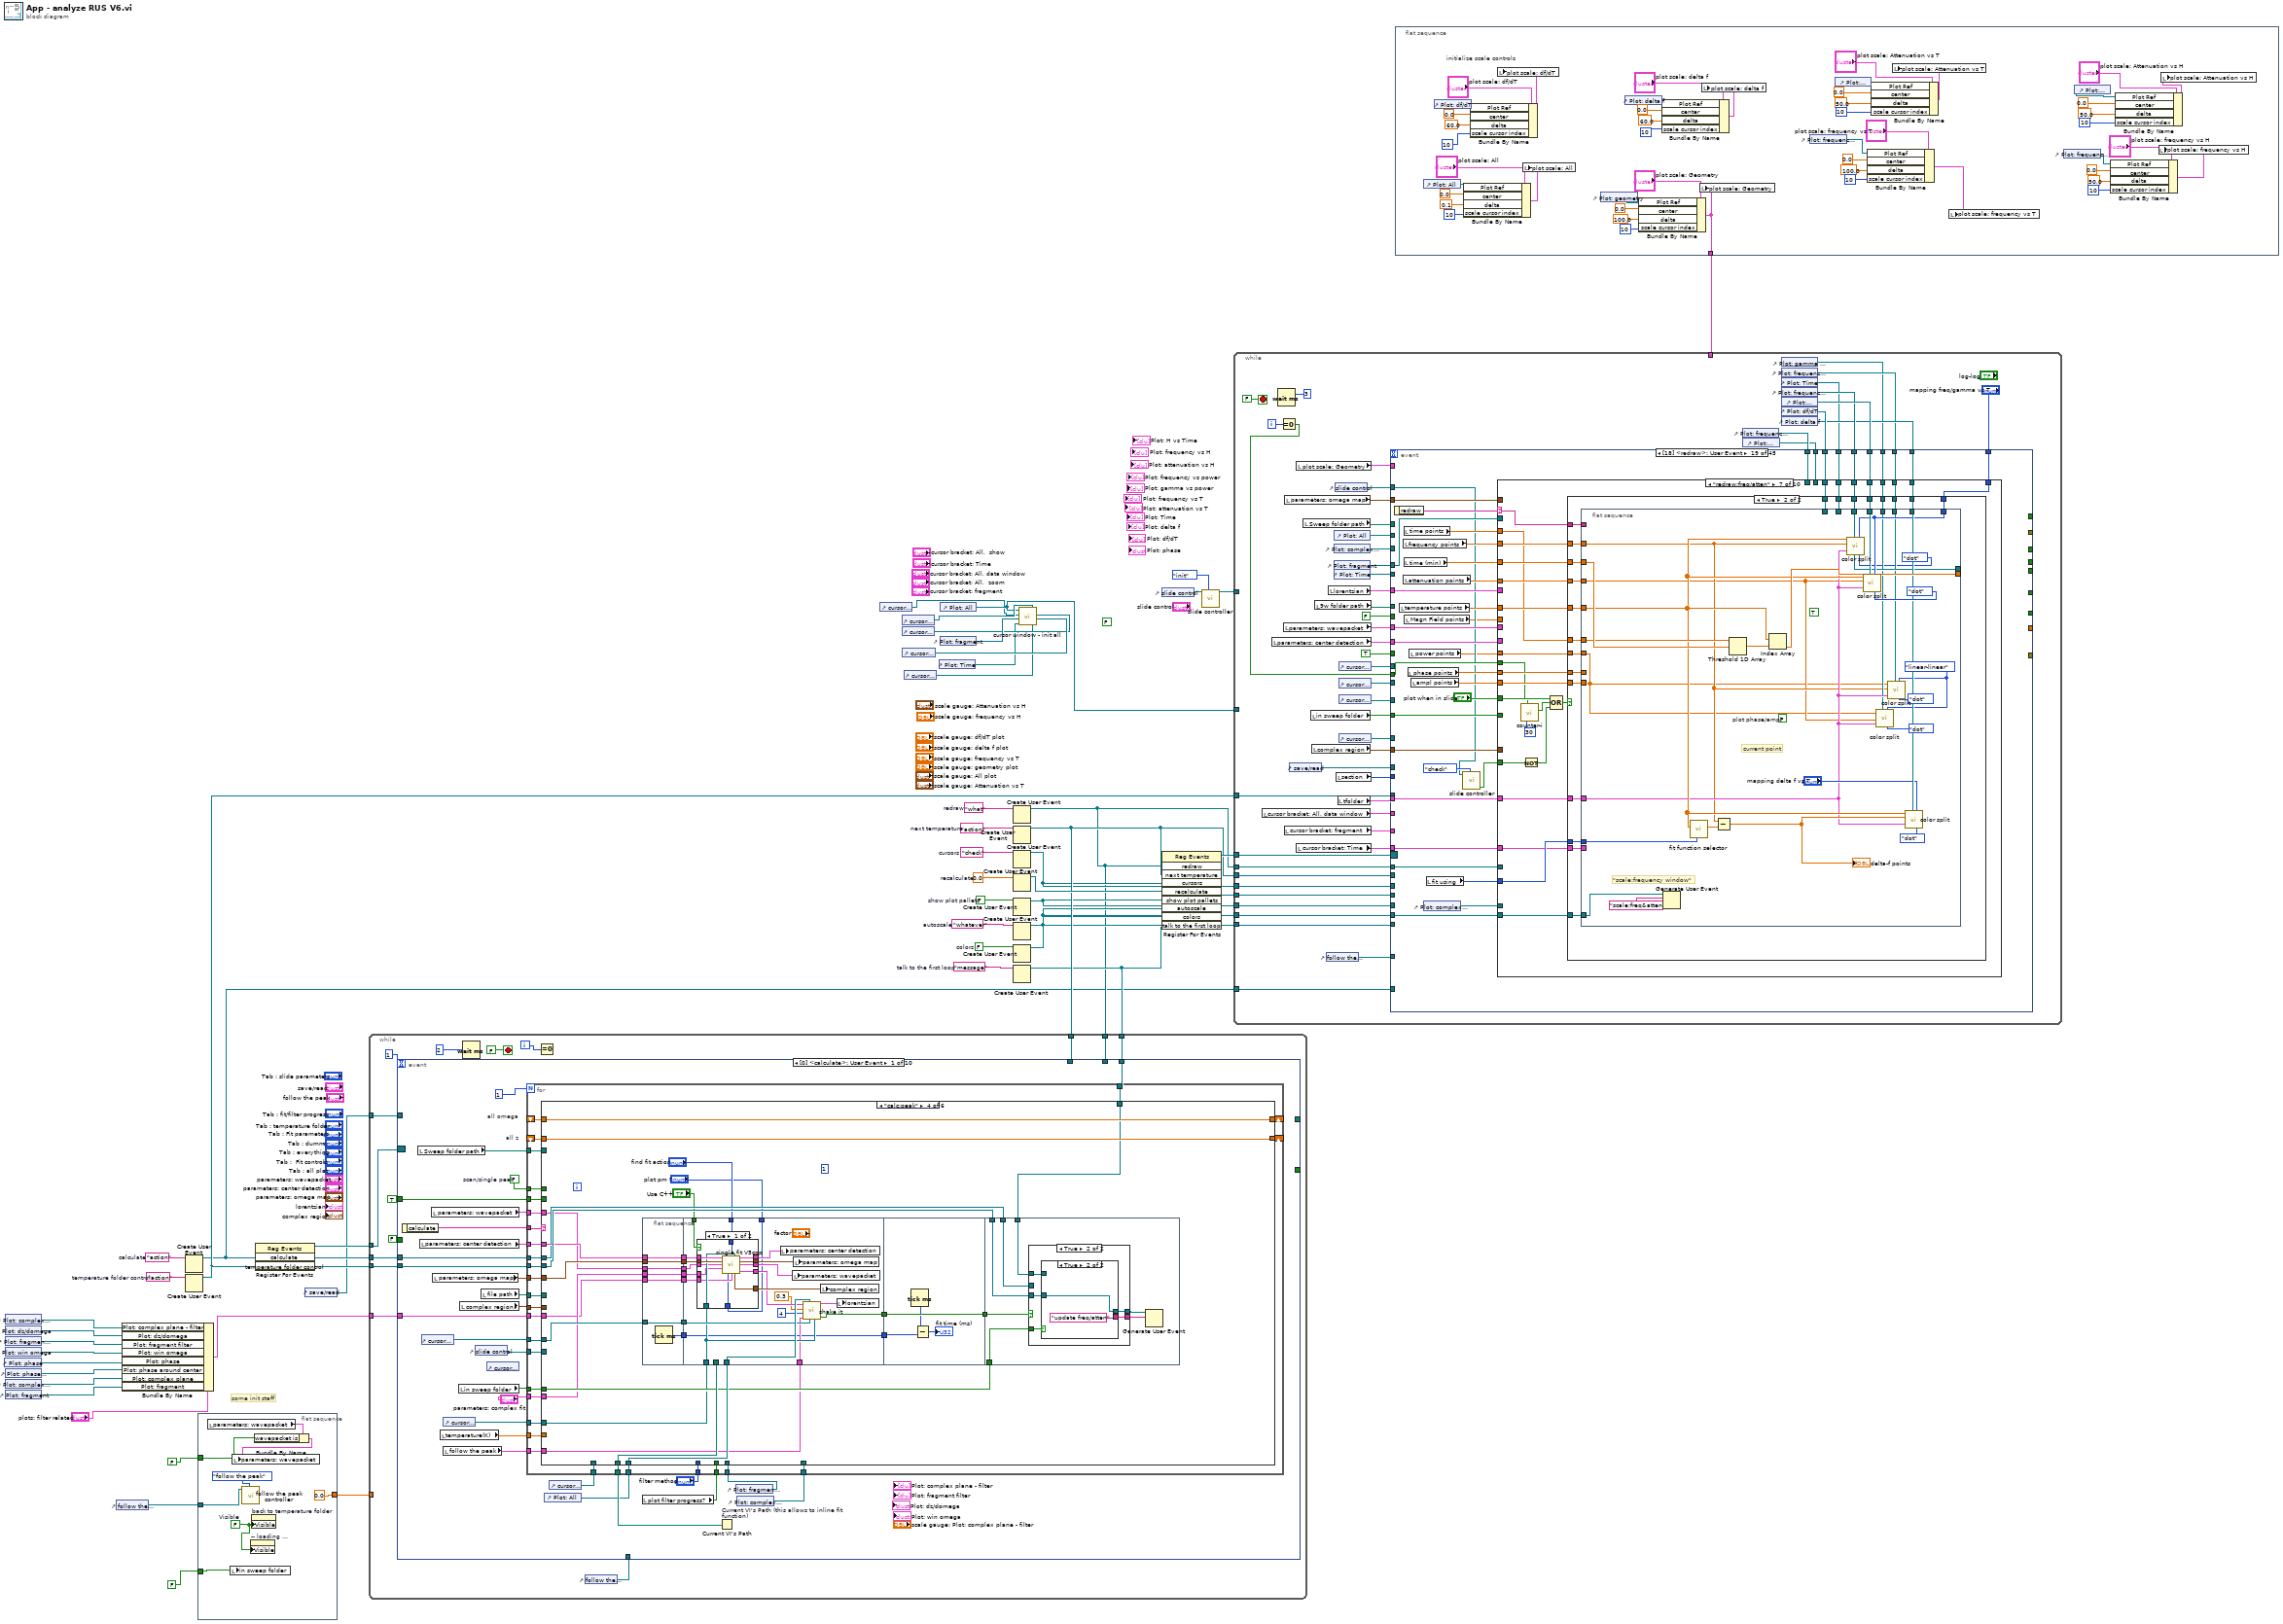
[diagram p0: block diagram]
diagram:
  (unwired) FALSE ("Boolean")
  w29 = "action"  # calculate
  w30 = "check"  # cursors
  w31 = "whatever"  # autoscale
  w32 = "what"  # redraw
  w34 = "message"  # talk to the first loop
  w35 = "action"  # temperature folder control
  w38 = FALSE  # colors
  w40 = FALSE  # show plot pallets
  w46 = 0.0  # recalculate
  w47 = "action"  # next temperature
  # "some init staff"
  n1 = control-ref of="Plot: phase"() -> (w7:refnum<vi>)
  n2 = control-ref of="Plot: complex plane - filter"() -> (w9:refnum<vi>)
  n3 = control-ref of="Plot: dz/domega"() -> (w10:refnum<vi>)
  n4 = control-ref of="Plot: fragment filter"() -> (w11:refnum<vi>)
  n5 = control-ref of="Plot: win omega"() -> (w8:refnum<vi>)
  n6 = control-ref of="Plot: phase around center"() -> (w13:refnum<vi>)
  n7 = control-ref of="Plot: complex plane"() -> (w12:refnum<vi>)
  n8 = control-ref of="Plot: fragment"() -> (w14:refnum<vi>)
  n9 = control-ref of="follow the peak"() -> (w5:refnum<vi>)
  n10 = Bundle By Name(cluster="plots: filter related", "Plot: complex plane - filter"=w9, "Plot: dz/domega"=w10, "Plot: fragment filter"=w11, "Plot: win omega"=w8, "Plot: phase"=w7, "Plot: phase around center"=w13, "Plot: complex plane"=w12, "Plot: fragment"=w14) -> (w6:T29)
  n11 = Create User Event(user event datatype=w29) -> (user event=w16:refnum<user-event>)  [unwired: 1 in, 1 out]
  n12 = Create User Event(user event datatype=w35) -> (user event=w18:refnum<user-event>)  [unwired: 1 in, 1 out]
  n13 = flat-sequence {
    tunnel: FALSE -> [w57]
    tunnel: FALSE -> [w52]
    tunnel: [0.0] -> w36
    tunnel: w5 -> [w50]
    frame #0 {
      w53 = FALSE  # Visible
      n14 = local read "parameters: wavepacket"() -> (w56:T16)
      n15 = local write "in sweep folder"(w57) -> ()
      n16 = call "follow the peak controller.vi"("action"=follow_the_peak_action."follow the peak", "follow the peak ref"=w50) -> ()  [unwired: 8 in, 2 out]
      n17 = property on="-- loading ..." class="Bool (strict)"("Visible"=w53) -> ()  [unwired: 2 in, 2 out]
      n18 = property on="back to temperature folder" class="Bool"("Visible"=w53) -> ()  [unwired: 2 in, 2 out]
      n19 = Bundle By Name(cluster=w56, "wavepacket is"=w52) -> (w55:T16)
      n20 = local write "parameters: wavepacket"(w55) -> ()
    }
  }
  n21 = register-events(w16, w18) -> (reference out=w48:refnum<event-registration>)  [unwired: 2 in, 1 out]
  n22 = control-ref of="save/read"() -> (w1:refnum<vi>)
  n23 = control-ref of="cursor bracket: All,  show"() -> (w19:refnum<vi>)
  n24 = control-ref of="cursor bracket: All, data window"() -> (w24:refnum<vi>)
  n25 = control-ref of="cursor bracket: All,  zoom"() -> (w23:refnum<vi>)
  n26 = control-ref of="cursor bracket: fragment"() -> (w25:refnum<vi>)
  n27 = control-ref of="cursor bracket: Time"() -> (w22:refnum<vi>)
  n28 = control-ref of="Plot: Time"() -> (w21:refnum<vi>)
  n29 = control-ref of="Plot: All"() -> (w20:refnum<vi>)
  n30 = control-ref of="Plot: fragment"() -> (w26:refnum<vi>)
  n31 = Create User Event(user event datatype=w34) -> (user event=w33:refnum<user-event>)  [unwired: 1 in, 1 out]
  n32 = Create User Event(user event datatype=w32) -> (user event=w17:refnum<user-event>)  [unwired: 1 in, 1 out]
  n33 = Create User Event(user event datatype=w47) -> (user event=w44:refnum<user-event>)  [unwired: 1 in, 1 out]
  n34 = while {
    tunnel: w48 -> [w72]
    tunnel: w16 -> [w70]
    tunnel: w44 -> [w69]
    tunnel: w36 -> [_]
    tunnel: w18 -> [w64]
    tunnel: w33 -> [w63]
    tunnel: w17 -> [w61]
    tunnel: w6 -> [w60]
    tunnel: w1 -> [w58]
    i -> [w62]
    stop <- FALSE stop-if-true
    n35 = Wait (ms)(milliseconds to wait=u32 2) -> ()  [unwired: 1 out]
    n36 = Equal To 0?(x=w62) -> ()  [unwired: 1 out]
    n37 = control-ref of="follow the peak"() -> (w59:refnum<vi>)
    n38 = event shown="[0] <calculate>: User Event" {
      selector: w72 -> [_ _ _ _ _ _ _ _ _ _]
      dyn-events: _ -> [_ _ _ _ _ _ _ _ _ _]
      timeout: 1 -> [_ _ _ _ _ _ _ _ _ _]
      tunnel: w70 -> [w98 w515 _ _ _ _ _ _ w1074 _]
      tunnel: w69 -> [_ _ _ _ _ _ _ _ _ _]
      tunnel: [_ _ _ "back to temperature folder" _ _ _ _ _ _] -> _
      tunnel: TRUE -> [w97 _ _ _ _ _ _ _ _ _]
      tunnel: FALSE -> [_ w517 _ _ w1054 _ _ _ _ _]
      tunnel: w64 -> [w100 w516 w1040 _ w1059 w1068 w1072 _ w1081 _]
      tunnel: [_ _ "Sweep folder path" _ _ _ _ _ _ _] -> _
      tunnel: w63 -> [w89 w513 _ _ _ _ _ _ _ _]
      tunnel: w61 -> [_ w491 w1038 _ _ _ _ _ _ _]
      tunnel: w60 -> [w75 _ _ _ _ _ _ _ _ _]
      tunnel: w59 -> [_ w488 _ _ _ _ _ _ _ _]
      tunnel: w58 -> [_ _ _ _ w1053 w1065 w1069 _ _ _]
      event User Event {
        w84 = FALSE  # scan/single peak
        # "all z"
        # "all omega"
        n39 = event-data() -> ("calculate"=w99:string)  [unwired: 1 in]
        n40 = local read "Sweep folder path"() -> (w81:path)
        n41 = local read "parameters: center detection"() -> (w91:T21)
